vi "Z6_Beamline_Chief.panel.vi"(0 "object ref":refnum<vi>, 5 "error in (no error)":errorcluster) -> (19 "error out":errorcluster)   [LabVIEW 2014, in "Z6_Beamline_Chief.lvlib"]
doc: "By this VI a hardware switch can be monitored and switched. \n\nThe indicators \"FALSE\", \"TRUE\" and \"SWITCH STATE\" show the value of the Beckhoff-Tag: blue indicates bad tag status reference problems, darkgreen false and lightgreen true. If everything is working fine, \"FALSE\" and \"SWITCH STATE\" should show the same value, while \"TRUE\" has the opposite value. The caption of the sensors for \"FALSE\" and \"TRUE\" are taken out of the database. In case of only one or no sensor these GUI elements are not shown at all.\n\nThe oval button switches. It should be in the same state as the \"SWITCH STATE\" indicator. \n\n\"Delete Instance\" disconnects and removes the instance from the PCS.\n\n\nLicense Agreement for this software:\n\nCopyright (C)\nGesellschaft für Schwerionenforschung, GSI\nPlanckstr. 1\n64291 Darmstadt\nGermany\n\nContact: D.Beck@gsi.de \n\nThis program is free software; you can redistribute it and/or modify it under the terms of the GNU General Public License as published by the Free Software Foundation; either version 2 of the license, or (at your option) any later version.\n\nThis program is distributed in the hope that it will be useful, but WITHOUT ANYW ARRANTY; without even the implied warranty of MERCHANTABILITY or FITNESS FOR A PARTICULAR PURPOSE. See the GNU General License for more details (http://www.gnu.org).\n\nGesellschaft für Schwerionenforschung, GSI\nPlanckstr. 1, 64291 Darmstadt, Germany\nFor all questions and ideas contact: M.Richter@gsi.de, H.Brand@gsi.de or D.Beck@gsi.de.\nLast update: 18-DEC-2002"
uses:
  Z6_Beamline_Chief.lvlib
  PH_Common/Picture/PH_Picture.GUI Element 36x36.ctl
  PH_Common/Picture/PH_Picture.GUI Element 24x36.ctl
  PH_Common/Picture/PH_Picture.GUI Element.ctl
  Z6_Beamline/Z6_Beamline.Switch Instances.ctl
  Z6_Beamline/Z6_Beamline.Black Box Instances.ctl
  PH_SystemInformation/PH_SystemInformation.GUI Refs.ctl
  PH_BL-Master/PH_BL-Master.GUI Refs.ctl
  Z6_Beamline/Z6_Beamline.GUI Refs.ctl
  Z6_Beamline/Z6_Beamline.Subsystem ok GUI Refs.ctl
  PH_Common/PH_Common.lvlib
  PH_BL-Master/PH_BL-Master.lvlib
  PH_SystemInformation/PH_SystemInformation.lvlib
  PH_Class/PH_Class.lvlib
  Z6_Beamline/Z6_Beamline.lvlib
panel:
  in  "Z6 Black Box Instances":T1="Z6_ST_Attenuator_1_BB"
  in  "Z6 Switch Instances":T2="Shutter_Exp4"
  out "Exp 3":u32(colorbox)
  out "Exp 2":u32(colorbox)
  out "Exp 1":u32(colorbox)
  out "Emergency Off":u32(colorbox)
  in  "Remote Desktop Connection":bool
  out "PHELIX_Timing_Mode":enum32{"10 Hz", "0.5 Hz", "Shot"}(radio) caption="Modeselector"
  in  "PCS System Indicator":bool caption="PCS"
  in  "CoG":bool
  in  "Calibrator":bool
  in  "Image Statistician":bool
  in  "Z6 Main":bool
  out "Exp 4 (Z6)":u32(colorbox)
  in  "Tab Control":T3(tab)
  out "PA_CH1_BB":T4 caption="CH"
  out "ns_WP_RR_6PWpGUI":T5 caption="Waveplate ns Frontend"
  out "YLF_WP_6PWpGUI":T5 caption="Waveplate YLF"
  out "fs_WP_Exit_6PWpGUI":T5 caption="Waveplate fs Frontend"
  in  "Hop 3":bool
  out "Frontends ok":bool caption="ok"
  out "MA_MM8_6PGUI":T6
  out "MA_MM9_6PGUI":T6
  out "MA_VacuumControl::MA_VacuumControl_Z6 Telescope BL Prepressure":dbl=2000.0 caption="mbar" format="%#_2e"
  out "BL-Z6-CH10":T4
  out "BL NT 2":u32(colorbox)
  out "BL-Z6-CH9":T4
  out "BL-Z6-Beamdump":bool=TRUE
  in  "Hop 4":bool
  out "Z6_SHG_TIP-TILT_6PGUI":T6
  out "Z6_SHG_ROT_6PGUI":T6
  out "MA_VacuumControl::MA_VacuumControl_Z6 Telescope BL":dbl=2000.0 caption="mbar" format="%#_2e"
  out "BL NT 3":u32(colorbox)
  out "Z6_MM10_6PGUI":T6
  in  "Hop 1":bool
  out "Shutter_Exp4":bool=TRUE
  in  "\"D:\\PCS\\Remote Access\\Z6-Northtower.rdp\"":bool caption="OK Button"
  out "Northtower ok":bool caption="ok"
  in  "\"D:\\PCS\\Remote Access\\Z6-Southtower.rdp\"":bool caption="OK Button"
  out "Southtower ok":bool caption="ok"
  in  "Z6_ST_Attenuator_1_BB":bool=TRUE
  out "Z6_ST_Attenuator_2_BB":T5 caption="BB 2"
  out "Z6_green_Alignment_Powermeter":bool=TRUE
  out "BL-Z6-CH11":T4
  out "Z6_ST_WP_6PWpGUI":T5 caption="Waveplate"
  in  "Hop 5":bool
  out "Z6_ST_NF_green_Cam":bool=TRUE caption="PA NF Exit Cam"
  out "Z6_green_Powermeter":bool=TRUE
  out "BL ST 10":u32(colorbox)
  out "BL ST 9":u32(colorbox)
  out "BL ST 8":u32(colorbox)
  out "BL ST 7":u32(colorbox)
  out "Z6_IR_Powermeter":bool=TRUE
  out "BL ST 6":u32(colorbox)
  out "Z6_ST_NF_IR_Cam":bool=TRUE caption="PA FF Exit Cam"
  out "BL ST 5":u32(colorbox)
  out "BL ST 4":u32(colorbox)
  out "BL ST 3":u32(colorbox)
  out "BL ST 1":u32(colorbox)
  in  "Hop 2":bool
  out "BL ST 2":u32(colorbox)
  out "Z6_MM11_6PGUI":T6
  out "Z6_ST_Flip_Cam_BB":T6
  out "Z6_ST_Flip_PD_BB":T6
  in  "\"D:\\PCS\\Remote Access\\Z6-Compressor.rdp\"":bool caption="OK Button"
  in  "Z6_ST_COS_Sensitivity_Switch_BB":bool=TRUE
  out "Z6_ST_COS_WP_6PWpGUI":T5 caption="Waveplate"
  out "Z6_ST_COS_Filt_1_BB":T5 caption="Filt 1"
  out "Z6_ST_COS_Filt_2_BB":bool=TRUE
  out "Z6_COS_Powermeter":bool=TRUE
  out "BL 100TW COS 6":u32(colorbox)
  out "BL 100TW COS 5":u32(colorbox)
  out "Z6_Compressor-SSAC":bool=TRUE
  out "Z6_COS_SSAC_Cam":bool=TRUE caption="PA NF Exit Cam"
  out "Z6_COS_NF_ImageOperator":bool=TRUE
  out "Z6_COS_NF_Cam":bool=TRUE caption="PA NF Exit Cam"
  out "Z6_COS_FF_Cam":bool=TRUE caption="PA FF Exit Cam"
  in  "Hop 6":bool
  out "100TW COS ok":bool caption="ok"
  out "Ready for Shot":bool
  out "MainAmp enabled":u32(colorbox)
  out "Laser enabled":u32(colorbox)
  out "PreAmp enabled":u32(colorbox)
  in  "Minimize":bool
  in  "Delete":bool
  out "loop counter":i32
  # "Z6-CS"
  # "3.40"
  # "2"
  # "1"
  # "GREEN"
  # "IR"
  # "1"
  # "2"
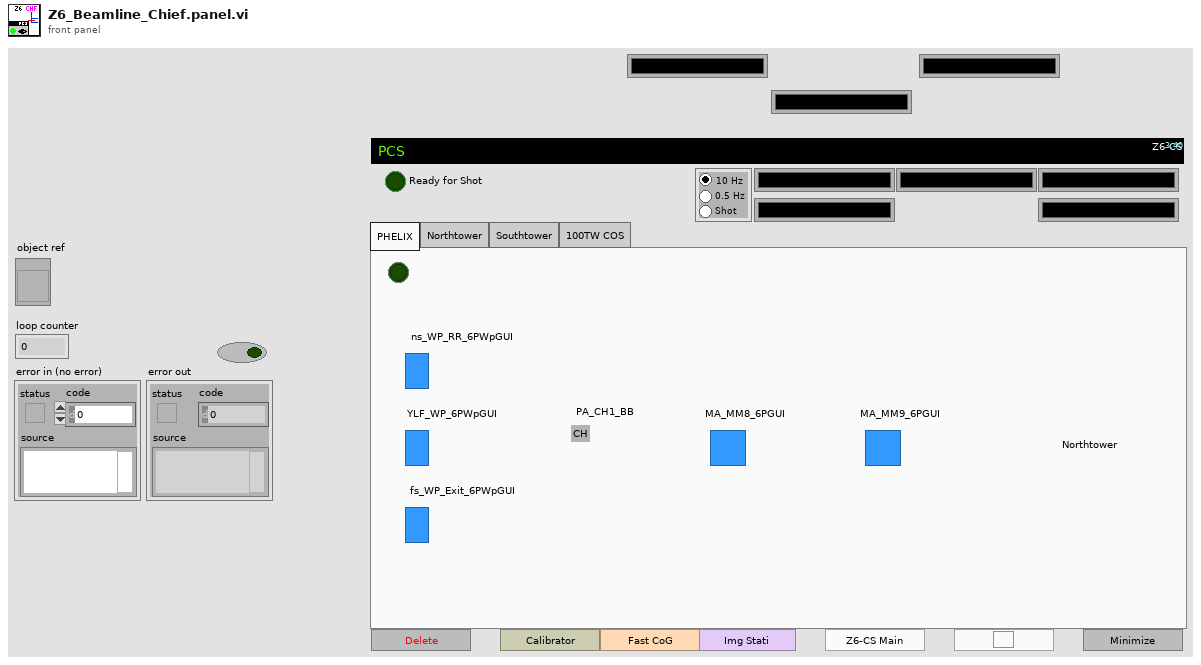
[diagram p1: front panel]
types:
  T1 = typedef "Z6_Beamline.lvlib/Z6_Beamline.Black Box Instances.ctl" = string
  T2 = typedef "Z6_Beamline.lvlib/Z6_Beamline.Switch Instances.ctl" = string
  T3 = enum32{"PHELIX", "Northtower", "Southtower", "100TW COS"}
  T4 = typedef "PH_Common.lvlib/PH_Picture.GUI Element.ctl" = picture
  T5 = typedef "PH_Common.lvlib/PH_Picture.GUI Element 24x36.ctl" = picture
  T6 = typedef "PH_Common.lvlib/PH_Picture.GUI Element 36x36.ctl" = picture
  T7 = typedef "Z6_Beamline.lvlib/Z6_Beamline.GUI Refs.ctl" = cluster{"BL NT":refnum<vi>[], "BL ST":refnum<vi>[], "BL 100 TW COS":refnum<vi>[], "Subs ok GUI Refs":T8}
  T8 = typedef "Z6_Beamline.lvlib/Z6_Beamline.Subsystem ok GUI Refs.ctl" = cluster{"Northtower ok":refnum<vi>, "Southtower ok":refnum<vi>, "Frontends ok":refnum<vi>, "100TW COS ok":refnum<vi>}
  T9 = typedef "PH_BL-Master.lvlib/PH_BL-Master.GUI Refs.ctl" = cluster{"Vac GUI Refs":refnum<vi>[], "O2 GUI Refs":refnum<vi>[], "Ready for Shot":refnum<vi>, "Boolean Condition Service Subscriber GUI Refs":refnum<vi>[], "Vision ID on same Node":string, "Picture Condition Service Subscriber GUI Refs":refnum<vi>[], "6P 4Q GUI Refs":refnum<vi>[], "Ref Switch GUI Instances":refnum<vi>, "Ref 6P Switch Instances":refnum<vi>, "Ref BB Instances":refnum<vi>, "Ref Switch Instances":refnum<vi>, "Ref Switch and 6P State Instances":refnum<vi>, "Boolean Status Service Subscriber GUI Refs":refnum<vi>[], "Picture Status Service Subscriber GUI Refs":refnum<vi>[], "Force Sensor Instances":refnum<vi>, "GUI Ref Delete":refnum<vi>}
  T10 = typedef "PH_SystemInformation.lvlib/PH_SystemInformation.GUI Refs.ctl" = cluster{"Laser":refnum<vi>, "PreAmp":refnum<vi>, "MainAmp":refnum<vi>, "Emergency Off":refnum<vi>, "Exp 1":refnum<vi>, "Exp 2":refnum<vi>, "Exp 3":refnum<vi>, "Exp 4":refnum<vi>, "Timing Mode GUI Ref":refnum<vi>}
  T11 = enum16{"PCS", "Laser", "Vision", "PP", "Special", "Beckhoff"}
  T12 = enum16{"None", "PCS Main", "Z6 Main", "PCS Beamline", "Z6 Beamline", "Image Statistician", "Powermeter Statistician", "SHS Anal Statistician", "Image Center of Gravity", "Image Calibrator", "SHS Analysis Calibrator", "Cam List", "Powermeterlist", "6P List", "BB List", "Switch List", "Sequence Watch"}
  T13 = typedef "PH_BL-Master.lvlib/PH_BL-Master.i attribute.ctl" = cluster{"Remote controlled":bool, "Boolean Condition Service Subscriber":refnum<vi>[], "Picture Condition Service Subscriber":refnum<vi>[], "R2S":cluster{"GUI Ref":refnum<vi>, "State":bool}, "Vacua":cluster{"GUI Ref":refnum<vi>, "Limit":dbl, "Curr Value":dbl, "in range":bool}[], "O2 Inspection":cluster{"GUI Ref":refnum<vi>, "Concentration":dbl, "State":T14}[], "Boolean Status Service Subscriber":cluster{"GUI Ref":refnum<vi>, "Status":T14, "no Link?":bool, "Status Subscriber Class":T15}[], "Picture Status Service Subscriber":cluster{"GUI Ref":refnum<vi>, "Status":T14, "no Link?":bool, "Status Subscriber Class":T15}[], "6P 4Q Service Subscriber":cluster{"GUI Ref":refnum<vi>, "Selector":T16, "no Link?":bool}[], "Index of latest 6P 4Q changing Instance":i32, "Index of latest Picture Status changing Instance":i32, "Index of latest Boolean Status changing Instance":i32, "Vision ID on same Node":string, "Start Phase over?":bool, "GUI Ref Delete":refnum<vi>}
  T14 = typedef "PH_StatusHandler.lvlib/PH_StatusHandler.Status.ctl" = i16
  T15 = typedef "PH_BL-Master.lvlib/PH_BL-Master.Status Subscriber Class.ctl" = enum16{"unknown", "Switch", "BB", "6P Switch", "Switch GUI", "Switch and 6P State", "Force Sensor"}
  T16 = typedef "PH_4_Pos_Selector.lvlib/PH_4_Pos_Selector.Position Selector.ctl" = u16
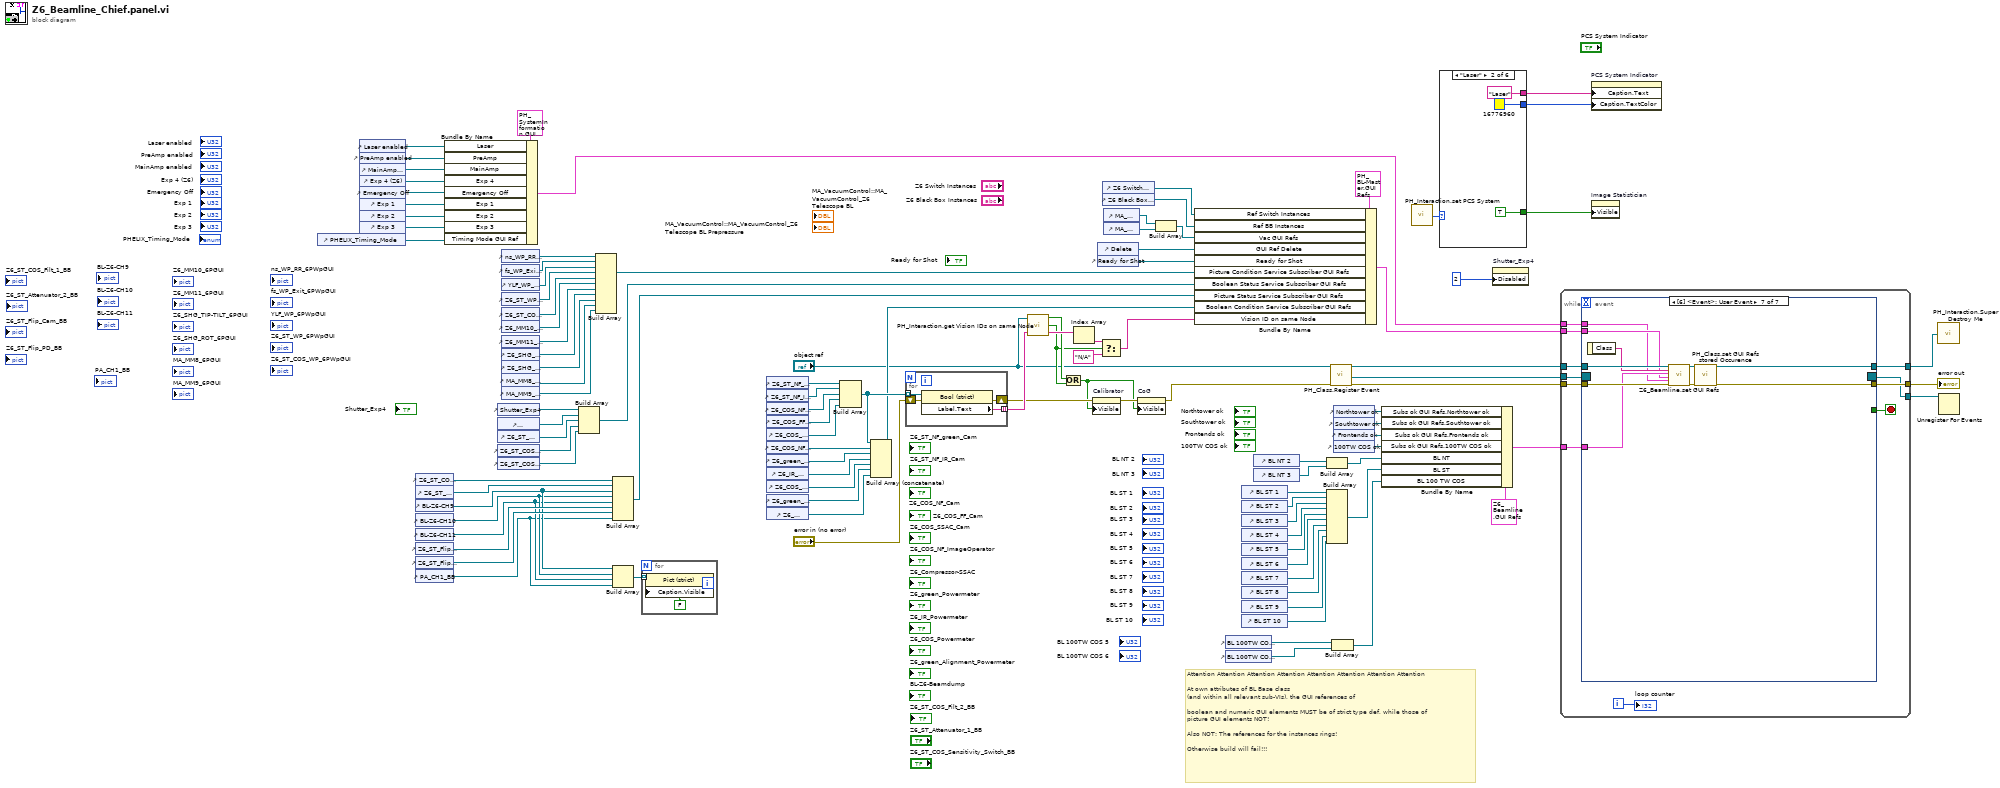
[diagram p0: block diagram]
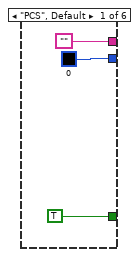
[diagram p2: hidden frame]
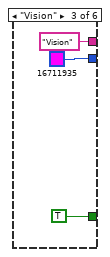
[diagram p3: hidden frame]
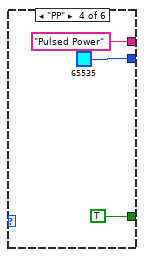
[diagram p4: hidden frame]
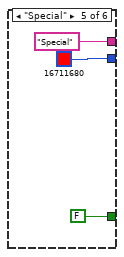
[diagram p5: hidden frame]
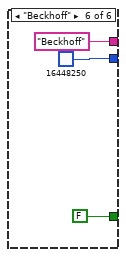
[diagram p6: hidden frame]
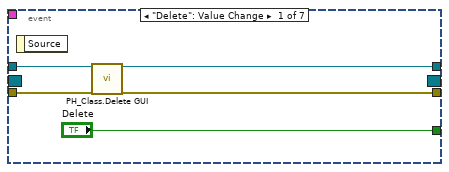
[diagram p7: hidden frame]
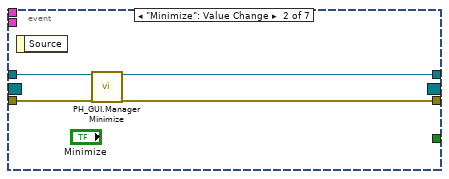
[diagram p8: hidden frame]
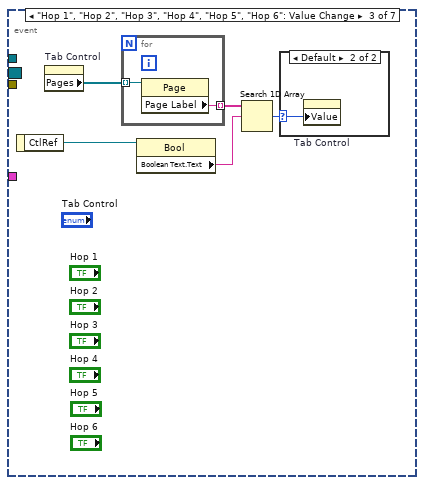
[diagram p9: hidden frame]
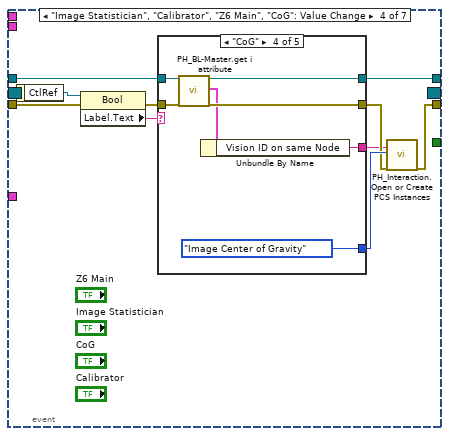
[diagram p11: hidden frame]
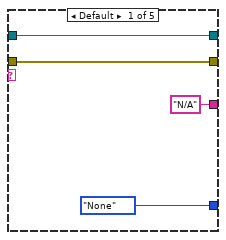
[diagram p12: hidden frame]
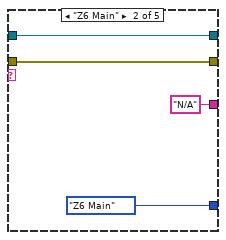
[diagram p13: hidden frame]
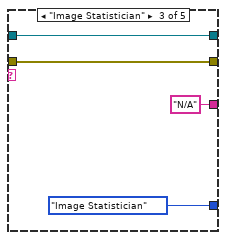
[diagram p14: hidden frame]
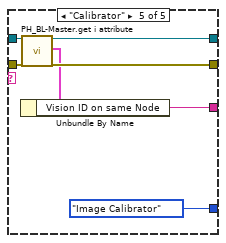
[diagram p15: hidden frame]
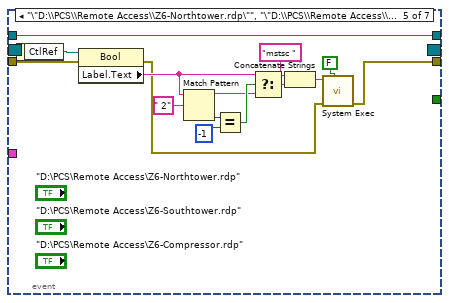
[diagram p16: hidden frame]
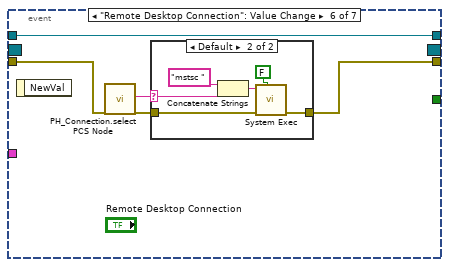
[diagram p17: hidden frame]
diagram:
  # "Attention Attention Attention Attention Attention Attention Attention Attention\n\nAt own attributes of BL Base class \n(and within all relevant sub-VIs), the GUI references of\n\nboolean and numeric GUI elements MUST be of strict type def, while those of\npicture GUI elements NOT!\n\nAlso NOT: The references for the instances rings!\n\nOtherwise build will fail!!!"
  n1 = control-ref of="PHELIX_Timing_Mode"() -> (w32:refnum<vi>)
  n2 = control-ref of="Laser enabled"() -> (w93:refnum<vi>)
  n3 = control-ref of="PreAmp enabled"() -> (w94:refnum<vi>)
  n4 = control-ref of="MainAmp enabled"() -> (w95:refnum<vi>)
  n5 = control-ref of="Exp 4 (Z6)"() -> (w96:refnum<vi>)
  n6 = control-ref of="Emergency Off"() -> (w67:refnum<vi>)
  n7 = control-ref of="Exp 1"() -> (w66:refnum<vi>)
  n8 = control-ref of="Exp 2"() -> (w65:refnum<vi>)
  n9 = control-ref of="Exp 3"() -> (w64:refnum<vi>)
  n10 = control-ref of="Z6_ST_COS_Filt_1_BB"() -> (w84:refnum<vi>)
  n11 = control-ref of="Z6_ST_Attenuator_2_BB"() -> (w83:refnum<vi>)
  n12 = control-ref of="BL-Z6-CH9"() -> (w71:refnum<vi>)
  n13 = control-ref of="BL-Z6-CH10"() -> (w70:refnum<vi>)
  n14 = control-ref of="BL-Z6-CH11"() -> (w69:refnum<vi>)
  n15 = control-ref of="Z6_ST_Flip_Cam_BB"() -> (w75:refnum<vi>)
  n16 = control-ref of="Z6_ST_Flip_PD_BB"() -> (w74:refnum<vi>)
  n17 = control-ref of="PA_CH1_BB"() -> (w52:refnum<vi>)
  n18 = Bundle By Name(cluster=T10 {"Laser"=refnum, "PreAmp"=refnum, "MainAmp"=refnum, "Emergency Off"=refnum, "Exp 1"=refnum, "Exp 2"=refnum, "Exp 3"=refnum, "Exp 4"=refnum, "Timing Mode GUI Ref"=refnum} ("System Information GUI Refs"), "Laser"=w93, "PreAmp"=w94, "MainAmp"=w95, "Exp 4"=w96, "Emergency Off"=w67, "Exp 1"=w66, "Exp 2"=w65, "Exp 3"=w64, "Timing Mode GUI Ref"=w32) -> (w2:T10)
  n19 = control-ref of="Shutter_Exp4"() -> (w62:refnum<vi>)
  n20 = control-ref of="BL-Z6-Beamdump"() -> (w61:refnum<vi>)
  n21 = control-ref of="Z6_ST_Attenuator_1_BB"() -> (w55:refnum<vi>)
  n22 = control-ref of="Z6_ST_COS_Sensitivity_Switch_BB"() -> (w54:refnum<vi>)
  n23 = control-ref of="Z6_ST_COS_Filt_2_BB"() -> (w53:refnum<vi>)
  n24 = control-ref of="ns_WP_RR_6PWpGUI"() -> (w82:refnum<vi>)
  n25 = control-ref of="fs_WP_Exit_6PWpGUI"() -> (w81:refnum<vi>)
  n26 = control-ref of="YLF_WP_6PWpGUI"() -> (w80:refnum<vi>)
  n27 = control-ref of="Z6_ST_WP_6PWpGUI"() -> (w79:refnum<vi>)
  n28 = control-ref of="Z6_ST_COS_WP_6PWpGUI"() -> (w78:refnum<vi>)
  n29 = control-ref of="Z6_MM10_6PGUI"() -> (w77:refnum<vi>)
  n30 = control-ref of="Z6_MM11_6PGUI"() -> (w76:refnum<vi>)
  n31 = control-ref of="Z6_SHG_ROT_6PGUI"() -> (w73:refnum<vi>)
  n32 = control-ref of="Z6_SHG_TIP-TILT_6PGUI"() -> (w72:refnum<vi>)
  n33 = control-ref of="MA_MM8_6PGUI"() -> (w35:refnum<vi>)
  n34 = control-ref of="MA_MM9_6PGUI"() -> (w34:refnum<vi>)
  n35 = Build Array(w62, w61, w55, w54, w53) -> (w20:refnum<vi>[])
  n36 = Build Array(w82, w81, w80, w79, w78, w77, w76, w73, w72, w35, w34) -> (w21:refnum<vi>[])
  n37 = Build Array(w84, w83, w71, w70, w69, w75, w74, w52) -> (w19:refnum<vi>[])
  n38 = Build Array(w71, w70, w69, w52) -> (w68:refnum<vi>[])
  n39 = for {
    tunnel: w68 -> [w109] mode=indexing
    n40 = property class="Pict (strict)"(reference=w109, "Caption.Visible"=FALSE) -> ()  [unwired: 1 in, 2 out]
  }
  n41 = control-ref of="Z6_ST_NF_green_Cam"() -> (w44:refnum<vi>)
  n42 = control-ref of="Z6_ST_NF_IR_Cam"() -> (w43:refnum<vi>)
  n43 = control-ref of="Z6_COS_NF_Cam"() -> (w42:refnum<vi>)
  n44 = control-ref of="Z6_COS_FF_Cam"() -> (w41:refnum<vi>)
  n45 = control-ref of="Z6_COS_SSAC_Cam"() -> (w40:refnum<vi>)
  n46 = control-ref of="Z6_COS_NF_ImageOperator"() -> (w63:refnum<vi>)
  n47 = control-ref of="Z6_green_Powermeter"() -> (w60:refnum<vi>)
  n48 = control-ref of="Z6_IR_Powermeter"() -> (w59:refnum<vi>)
  n49 = control-ref of="Z6_COS_Powermeter"() -> (w58:refnum<vi>)
  n50 = control-ref of="Z6_green_Alignment_Powermeter"() -> (w57:refnum<vi>)
  n51 = control-ref of="Z6_Compressor-SSAC"() -> (w56:refnum<vi>)
  n52 = Build Array(w44, w43, w42, w41, w40) -> (w39:refnum<vi>[])
  n53 = Build Array (concatenate)(w39, w63, w60, w59, w58, w57, w56) -> (w13:refnum<vi>[])
  n54 = for {
    shift-right: [w112] -> w17
    shift-left: "error in (no error)" -> [w113]
    tunnel: [w111] -> w47 mode=indexing
    tunnel: w39 -> [w110] mode=indexing
    n55 = property class="Bool (strict)"(reference=w110, error in=w113) -> (error out=w112:errorcluster, "Label.Text"=w111:string)  [unwired: 1 out]
  }
  n56 = call "PH_Interaction.get Vision IDs on same Node.vi"("Cam Instances"=w47, "i ref in"="object ref") -> ("Vision System IDs"=w38:string[], "Vision Sytem IDs found"=w36:bool, "Cams instanciated on own system"=w37:bool)  [unwired: 1 in]
  n57 = Or(x=w37, y=w36) -> (x .or. y?=w16:bool)
  n58 = Index Array(array=w38) -> (element=w46:string)  [unwired: 1 in]
  n59 = property on="Calibrator" class="Bool"(error in=w17, "Visible"=w16) -> (error out=w18:errorcluster)  [unwired: 1 in, 1 out]
  n60 = control-ref of="Delete"() -> (w1:refnum<vi>)
  n61 = control-ref of="Ready for Shot"() -> (w22:refnum<vi>)
  n62 = Select(t=w46, s=w36, f="N/A") -> (s? t:f=w14:string)
  n63 = control-ref of="Z6 Switch Instances"() -> (w25:refnum<vi>)
  n64 = control-ref of="Z6 Black Box Instances"() -> (w24:refnum<vi>)
  n65 = control-ref of="MA_VacuumControl::MA_VacuumControl_Z6 Telescope BL"() -> (w102:refnum<vi>)
  n66 = control-ref of="MA_VacuumControl::MA_VacuumControl_Z6 Telescope BL Prepressure"() -> (w33:refnum<vi>)
  n67 = property on="CoG" class="Bool"(error in=w18, "Visible"=w16) -> (error out=w15:errorcluster)  [unwired: 1 in, 1 out]
  n68 = Build Array(w102, w33) -> (w23:refnum<vi>[])
  n69 = Bundle By Name(cluster=T9 {"Vac GUI Refs"=[], "O2 GUI Refs"=[], "Ready for Shot"=refnum, "Boolean Condition Service Subscriber GUI Refs"=[], "Vision ID on same Node"="", "Picture Condition Service Subscriber GUI Refs"=[], "6P 4Q GUI Refs"=[], "Ref Switch GUI Instances"=refnum, "Ref 6P Switch Instances"=refnum, "Ref BB Instances"=refnum, "Ref Switch Instances"=refnum, "Ref Switch and 6P State Instances"=refnum, "Boolean Status Service Subscriber GUI Refs"=[], "Picture Status Service Subscriber GUI Refs"=[], "Force Sensor Instances"=refnum, "GUI Ref Delete"=refnum} ("PH_BL_Master GUI Refs"), "Ref Switch Instances"=w25, "Ref BB Instances"=w24, "Vac GUI Refs"=w23, "GUI Ref Delete"=w1, "Ready for Shot"=w22, "Picture Condition Service Subscriber GUI Refs"=w21, "Boolean Status Service Subscriber GUI Refs"=w20, "Picture Status Service Subscriber GUI Refs"=w19, "Boolean Condition Service Subscriber GUI Refs"=w13, "Vision ID on same Node"=w14) -> (w3:T9)
  n70 = control-ref of="BL 100TW COS 5"() -> (w99:refnum<vi>)
  n71 = control-ref of="BL 100TW COS 6"() -> (w98:refnum<vi>)
  n72 = control-ref of="BL ST 1"() -> (w101:refnum<vi>)
  n73 = control-ref of="BL ST 2"() -> (w100:refnum<vi>)
  n74 = control-ref of="BL ST 3"() -> (w92:refnum<vi>)
  n75 = control-ref of="BL ST 4"() -> (w91:refnum<vi>)
  n76 = control-ref of="BL ST 5"() -> (w90:refnum<vi>)
  n77 = control-ref of="BL ST 6"() -> (w89:refnum<vi>)
  n78 = control-ref of="BL ST 7"() -> (w88:refnum<vi>)
  n79 = control-ref of="BL ST 8"() -> (w87:refnum<vi>)
  n80 = control-ref of="BL ST 9"() -> (w86:refnum<vi>)
  n81 = control-ref of="BL ST 10"() -> (w85:refnum<vi>)
  n82 = control-ref of="BL NT 2"() -> (w106:refnum<vi>)
  n83 = control-ref of="BL NT 3"() -> (w105:refnum<vi>)
  n84 = Build Array(w106, w105) -> (w9:refnum<vi>[])
  n85 = Build Array(w101, w100, w92, w91, w90, w89, w88, w87, w86, w85) -> (w7:refnum<vi>[])
  n86 = call "PH_Class.Register Event.vi"("i ref in"="object ref", "error in (no error)"=w15) -> ("i ref out"=w30:refnum<vi>, "Event Registration Refnum"=w29:refnum<event-registration>, "error out"=w31:errorcluster)  [unwired: 15 in]
  n87 = Build Array(w99, w98) -> (w6:refnum<vi>[])
  n88 = control-ref of="Northtower ok"() -> ()  [unwired: 1 out]
  n89 = control-ref of="Southtower ok"() -> (w11:refnum<vi>)
  n90 = control-ref of="Frontends ok"() -> (w10:refnum<vi>)
  n91 = control-ref of="100TW COS ok"() -> (w8:refnum<vi>)
  n92 = Bundle By Name(cluster=T7 {"BL NT"=[], "BL ST"=[], "BL 100 TW COS"=[], "Subs ok GUI Refs"={"Northtower ok"=refnum, "Southtower ok"=refnum, "Frontends ok"=refnum, "100TW COS ok"=refnum}} ("GUI Refs"), "Subs ok GUI Refs.Northtower ok"=w11, "Subs ok GUI Refs.Southtower ok"=w10, "Subs ok GUI Refs.Frontends ok"=w8, "Subs ok GUI Refs.100TW COS ok"=w8, "BL NT"=w9, "BL ST"=w7, "BL 100 TW COS"=w6) -> (w12:T7)
  n93 = call "PH_Interaction.set PCS System.vi"() -> ("Enum"=w51:T11)  [unwired: 1 in]
  n94 = case shown="\"Laser\"" w51 {
    tunnel: ["" "Laser" "Vision" "Pulsed Power" "Special" "Beckhoff"] -> w50
    tunnel: [TRUE TRUE TRUE TRUE FALSE FALSE] -> w48
    tunnel: [u32 0 ("Color Box") u32 16776960 ("Color Box") u32 16711935 ("Color Box") u32 65535 ("Color Box") u32 16711680 ("Color Box") u32 16448250 ("Color Box")] -> w49
    frame "PCS", Default {
    }
    frame "Laser" {
    }
    frame "Vision" {
    }
    frame "PP" {
    }
    frame "Special" {
    }
    frame "Beckhoff" {
    }
  }
  n95 = property on="Shutter_Exp4" class="Bool (strict)"("Disabled"=u8 2) -> ()  [unwired: 2 in, 2 out]
  n96 = while {
    tunnel: w30 -> [w139]
    tunnel: [w138] -> w104
    tunnel: w31 -> [w141]
    tunnel: [w140] -> w103
    tunnel: w29 -> [w136]
    tunnel: [w135] -> w28
    tunnel: w12 -> [w134]
    tunnel: w3 -> [w133]
    tunnel: w2 -> [w132]
    i -> [w142]
    stop <- w137 stop-if-true
    n97 = event shown="[6] <Event>: User Event" {
      selector: w136 -> [_ _ _ _ _ _ _]
      dyn-events: [_ _ _ _ _ _ _] -> w135
      timeout: _ -> [_ _ _ _ _ _ _]
      tunnel: w139 -> [w147 w151 _ w162 w198 w212 w232]
      tunnel: w141 -> [w145 w150 _ w169 w209 w213 w231]
      tunnel: [w143 w149 _ w168 w199 w211 w229] -> w140
      tunnel: [w144 w148 _ w161 w198 w212 w227] -> w138
      tunnel: ["Delete" _ _ _ _ _ _] -> w137
      tunnel: w134 -> [_ _ _ _ _ _ w225]
      tunnel: w133 -> [_ _ _ _ _ _ w224]
      tunnel: w132 -> [_ _ _ _ _ _ w223]
      event "Delete": Value Change {
        n98 = event-data() -> ()  [unwired: 1 in, 1 out]
        n99 = call "PH_Class.Delete GUI.vi"("VI in"=w147, "error in (no error)"=w145) -> ("VI out"=w144:refnum<vi>, "error out"=w143:errorcluster)  [unwired: 16 in]
      }
      event "Minimize": Value Change {
        n100 = event-data() -> ()  [unwired: 1 in, 1 out]
        n101 = call "PH_GUI.Manager Minimize.vi"("i ref in"=w151, "error in"=w150) -> ("i ref out"=w148:refnum<vi>, "error out"=w149:errorcluster)  [unwired: 16 in]
      }
      event "Hop 1", "Hop 2", "Hop 3", "Hop 4", "Hop 5", "Hop 6": Value Change {
        n102 = event-data() -> ("CtlRef"=w156:refnum<vi>)  [unwired: 1 in]
        n103 = property on="Tab Control" class="TabCtl (strict)"() -> ("Pages"=w152:refnum<vi>[])  [unwired: 2 in, 2 out]
        n104 = for {
          tunnel: [w159] -> w155 mode=indexing
          tunnel: w152 -> [w158] mode=indexing
          n105 = property class="Page"(reference=w158) -> ("Page Label"=w159:string)  [unwired: 1 in, 2 out]
        }
        n106 = property class="Bool"(reference=w156) -> ("Boolean Text.Text"=w154:string)  [unwired: 1 in, 2 out]
        n107 = Search 1D Array(1D array=w155, element=w154) -> (index of element=w153:i32)  [unwired: 1 in]
        n108 = case shown="Default" w153 {
          selector: w153 -> [_ w157]
          frame -1 {
          }
          frame Default {
            n109 = property on="Tab Control" class="TabCtl (strict)"("Value"=w157) -> ()  [unwired: 2 in, 2 out]
          }
        }
      }
      event "Image Statistician", "Calibrator", "Z6 Main", "CoG": Value Change {
        n110 = event-data() -> ("CtlRef"=w167:refnum<vi>)  [unwired: 1 in]
        n111 = property class="Bool"(reference=w167, error in=w169) -> (error out=w164:errorcluster, "Label.Text"=w165:string)  [unwired: 1 out]
        n112 = case shown="\"CoG\"" w165 {
          tunnel: [T12."None" ("Instance to create or open") T12."Z6 Main" ("Instance to create or open") T12."Image Statistician" ("Instance to create or open") T12."Image Center of Gravity" ("Instance to create or open") T12."Image Calibrator" ("Instance to create or open")] -> w166
          tunnel: w164 -> [w171 w175 w179 w186 w194]
          tunnel: [w171 w175 w179 w184 w193] -> w163
          tunnel: w162 -> [w172 w176 w180 w187 w192]
          tunnel: [w172 w176 w180 w185 w191] -> w161
          tunnel: ["N/A" ("Vision ID on same Node") "N/A" ("Vision ID on same Node") "N/A" ("Vision ID on same Node") w182 w189] -> w160
          frame Default {
          }
          frame "Z6 Main" {
          }
          frame "Image Statistician" {
          }
          frame "CoG" {
            n113 = call "PH_BL-Master.get i attribute.vi"("i ref in"=w187, "error in (no error)"=w186) -> ("i ref out"=w185:refnum<vi>, "i attribute"=w183:T13, "error out"=w184:errorcluster)  [unwired: 15 in]
            n114 = Unbundle By Name(w183) -> ("Vision ID on same Node"=w182:string)
          }
          frame "Calibrator" {
            n115 = call "PH_BL-Master.get i attribute.vi"("i ref in"=w192, "error in (no error)"=w194) -> ("i ref out"=w191:refnum<vi>, "i attribute"=w190:T13, "error out"=w193:errorcluster)  [unwired: 15 in]
            n116 = Unbundle By Name(w190) -> ("Vision ID on same Node"=w189:string)
          }
        }
        n117 = call "PH_Interaction.Open or Create PCS Instances.vi"("System ID (N/A)"=w160, "Instance to create or open"=w166, "error IO"=w163) -> ("error out"=w168:errorcluster)  [unwired: 16 in]
      }
      event "\"D:\\PCS\\Remote Access\\Z6-Northtower.rdp\"", "\"D:\\PCS\\Remote Access\\Z6-Southtower.rdp\"", "\"D:\\PCS\\Remote Access\\Z6-Compressor.rdp\"": Value Change {
        n118 = event-data() -> ("CtlRef"=w210:refnum<vi>)  [unwired: 1 in]
        n119 = property class="Bool"(reference=w210, error in=w209) -> (error out=w196:errorcluster, "Label.Text"=w197:string)  [unwired: 1 out]
        n120 = Match Pattern(string=w197, regular expression=" 2") -> (before substring=w200:string, offset past match=w204:i32)  [unwired: 1 in, 2 out]
        n121 = Equal?(x=w204, y=-1) -> (x = y?=w202:bool)
        n122 = Select(t=w197, s=w202, f=w200) -> (s? t:f=w201:string)
        n123 = Concatenate Strings("mstsc " ("command line"), w201) -> (w207:string)
        n124 = call <vilib>:"System Exec.vi"("wait until completion? (T)"=FALSE, "error in (no error)"=w196, "command line"=w207) -> ("error out"=w199:errorcluster)  [unwired: 5 in, 3 out]
      }
      event "Remote Desktop Connection": Value Change {
        n125 = event-data() -> ()  [unwired: 1 in, 1 out]
        n126 = call "PH_Connection.select PCS Node.vi"("error in"=w213) -> ("string out"=w215:string, "error out"=w214:errorcluster)  [unwired: 17 in]
        n127 = case shown="Default" w215 {
          selector: w215 -> [_ w217]
          tunnel: w214 -> [w216 w219]
          tunnel: [w216 w218] -> w211
          frame "", "N/A" {
          }
          frame Default {
            n128 = Concatenate Strings("mstsc " ("command line"), w217) -> (w221:string)
            n129 = call <vilib>:"System Exec.vi"("wait until completion? (T)"=FALSE, "error in (no error)"=w219, "command line"=w221) -> ("error out"=w218:errorcluster)  [unwired: 5 in, 3 out]
          }
        }
      }
      event User Event {
        n130 = event-data() -> ("Class"=w226:string)  [unwired: 1 in]
        n131 = call "Z6_Beamline.set GUI Refs.vi"("VI in"=w232, "Class"=w226, "Z6 Beamline GUI Refs"=w225, "PH_BL_Master GUI Refs"=w224, "System Information GUI Refs"=w223, "error in (no error)"=w231) -> ("VI out"=w228:refnum<vi>, "error out"=w230:errorcluster)  [unwired: 12 in]
        n132 = call "PH_Class.set GUI Refs stored Occurence.vi"("i ref in"=w228, "error in (no error)"=w230) -> ("i ref out"=w227:refnum<vi>, "error out"=w229:errorcluster)  [unwired: 16 in]
      }
    }
    "loop counter" <- w142
  }
  "error out" <- w103
  n133 = property on="PCS System Indicator" class="Bool (strict)"("Caption.Text"=w50, "Caption.TextColor"=w49) -> ()  [unwired: 2 in, 2 out]
  n134 = property on="Image Statistician" class="Bool"("Visible"=w48) -> ()  [unwired: 2 in, 2 out]
  n135 = call "PH_Interaction.Super Destroy Me.vi"("i ref out"=w104) -> ()
  n136 = Unregister For Events(event registration refnum=w28) -> ()  [unwired: 1 in, 1 out]
